vi "New multiple timed message.vi"(6 "Repeats":i16=1, 7 "Target Queue":enum16{"Message", "Comms"}(ring), 8 "Period (ms)":u32, 9 "Data":variant, 10 "Message":string, 11 "RT Queues":T1) -> (1 "Schedule ID":u32, 3 "RT Queues out":T1)   [LabVIEW 2018, in "Message scheduler.lvlib"]
uses:
  Message scheduler.lvlib
  Type Defs/scheduled message cluster.ctl
  Type Defs/Queues cluster.ctl
  Chris VIs/Message Scheduler/message scheduler.lvclass
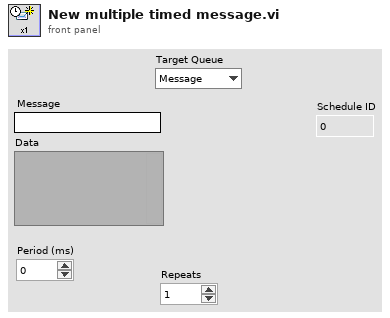
[diagram p1: front panel]
types:
  T1 = typedef "Queues cluster.ctl" = cluster{"RT Message":refnum<queue>, "RT Comms":refnum<queue>, "RT Data":refnum<queue>, "RT FIFO":refnum<queue>, "message scheduler":refnum<class "message scheduler.lvclass">}
  T2 = typedef "Message scheduler.lvlib/scheduled message cluster.ctl" = cluster{"message element":cluster{"Message":string, "Data":variant}, "schedule":cluster{"Repeats":i16, "Period (ms)":u32, "ID":u32, "Queue":enum16{"Message", "Comms"}, "T0":u32}, "Action":enum16{"New", "Remove", "Quit"}}
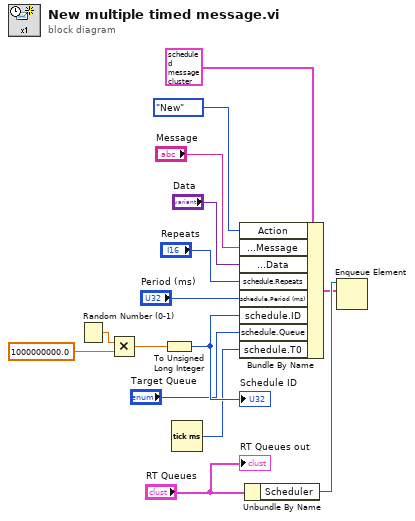
[diagram p0: block diagram]
diagram:
  n1 = Random Number (0-1)() -> (number: 0 to 1=w6:dbl)
  n2 = Multiply(x=w6, y=1000000000.0) -> (x*y=w4:dbl)
  n3 = To Unsigned Long Integer(number=w4) -> (unsigned 32bit integer=w3:u32)
  "Schedule ID" <- w3
  n4 = Tick Count (ms)() -> (millisecond timer value=w1:u32)
  n5 = Bundle By Name(cluster=T2 {"message element"={"Message"="", "Data"=variant}, "schedule"={"Repeats"=0, "Period (ms)"=0, "ID"=0, "Queue"=enum."Message", "T0"=0}, "Action"=enum."New"} ("Scheduled message"), "Action"=enum16{"New", "Remove", "Quit"}."New", "message element.Message"="Message", "message element.Data"="Data", "schedule.Repeats"="Repeats", "schedule.Period (ms)"="Period (ms)", "schedule.ID"=w3, "schedule.Queue"="Target Queue", "schedule.T0"=w1) -> (w12:T2)
  n6 = Unbundle By Name("RT Queues") -> ("Scheduler"=w14:refnum<queue>)
  n7 = Enqueue Element(queue=w14, element=w12) -> ()  [unwired: 2 in, 3 out]
  "RT Queues out" <- "RT Queues"
